vi "Mcp2210 Reset.vi"(8 "error in (no error)":errorcluster, 11 "handle":i32) -> (0 "error out":errorcluster, 3 "handle out":u32)   [LabVIEW 2015, in "mcp2210.lvlib"]
doc: "Reset the USB device.\nIn case of successful execution, the function closes the device handle and returns 0 (E_SUCCESS).\nIn case of failure, negative error code is returned.\n!!! Important note !!!\nThe user application must take into account the time needed for the device reset and for\nthe USB enumeration process. Trying to open the device too soon after reset may fail.\nPlease mind also that the time needed for USB enumeration may be different on different systems, and\nmay vary also on the same system, depending on the configuration, CPU load a.s.o.\nParameters:\nInputs:\n- void *handle - The pointer to the USB device handle. Cannot be NULL.\nOutputs:\n- none\nReturns:\n- 0 for success: E_SUCCESS\n- negative error code: E_ERR_NULL, E_ERR_INVALID_HANDLE_VALUE\nE_ERR_HID_TIMEOUT, E_ERR_HID_RW_FILEIO, E_ERR_UNKOWN_ERROR\nE_ERR_CLOSE_FAILED\n\nMCP2210_DLL_UM_API int __stdcall Mcp2210_Reset(void *handle);"
uses:
  <userlib>/mcp2210/mcp2210.lvlib
  <userlib>/mcp2210/mcp2210_dll_um_x86.dll
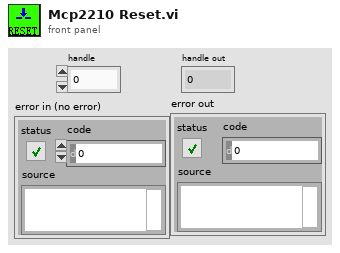
[diagram p1: front panel]
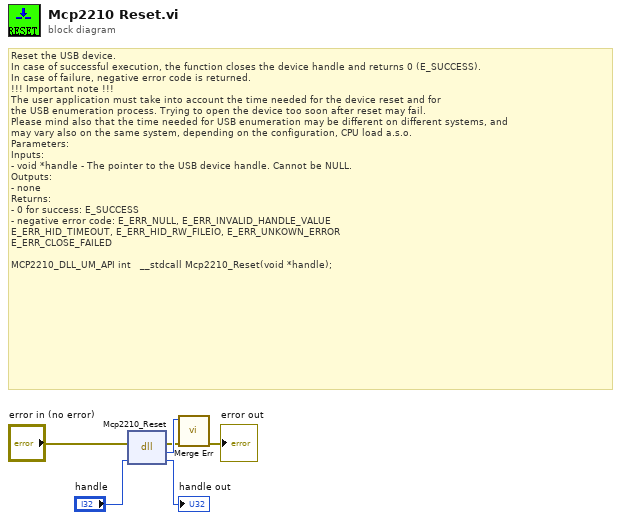
[diagram p0: block diagram]
diagram:
  # "Reset the USB device.\nIn case of successful execution, the function closes the device handle and returns 0 (E_SUCCESS).\nIn case of failure, negative error code is returned.\n!!! Important note !!!\nThe user application must take into account the time needed for the device reset and for\nthe USB enumeration process. Trying to open the device too soon after reset may fail.\nPlease mind also that the time needed for USB enumeration may be different on different systems, and\nmay vary also on the same system, depending on the configuration, CPU load a.s.o.\nParameters:\nInputs:\n- void *handle - The pointer to the USB device handle. Cannot be NULL.\nOutputs:\n- none\nReturns:\n- 0 for success: E_SUCCESS\n- negative error code: E_ERR_NULL, E_ERR_INVALID_HANDLE_VALUE\nE_ERR_HID_TIMEOUT, E_ERR_HID_RW_FILEIO, E_ERR_UNKOWN_ERROR\nE_ERR_CLOSE_FAILED\n\nMCP2210_DLL_UM_API int   __stdcall Mcp2210_Reset(void *handle);"
  n1 = dll-call lib="D:/LabVIEW 2015/user.lib/mcp2210/mcp2210_dll_um_x86.*" fn="Mcp2210_Reset"(error in="error in (no error)", "handle"="handle") -> (error out=w3:errorcluster, "return type"=w4:i32, "handle"=→"handle out":i32)  [unwired: 2 in, 1 out]
  n2 = call <userlib>:"Merge Err.vi"("error in (no error)"=w3, "return type"=w4) -> ("error out"=→"error out":errorcluster)  [unwired: 9 in]
